vi "Terminate.vi"(8 "error in (no error)":errorcluster, 10 "Message in":refnum<class "TerminateMessage.lvclass">, 11 "Galvo in":refnum<class "ImagingModeSPIM.lvclass">) -> (0 "error out":errorcluster, 3 "Galvo out":refnum<class "ImagingModeSPIM.lvclass">)   [LabVIEW 2012, in "ImagingModeSPIM.lvclass"]
doc: "This member function is called when the statemachine in the run.vi receives an 'terminate' command. It closes the RabbitMQ connection. \n\nOverride this member function in your derived class to release all previously acquired resources (but don't forget to call the parent method). If your component has subcomponents, they count as resources, and you have to release them by calling their own terminate functions."
uses:
  ImagingModeSPIM.lvclass
  <vilib>/Distrio/Murmex/TerminateMessage/TerminateMessage.lvclass
  ImagingModeSPIM.lvclass/ImagingModeSPIM.ctl
  <vilib>/Distrio/Murmex/Murmex/Murmex.lvclass
panel:
  # "This method is called when the TERMINATE\ntrigger is sent. \n\nOverride this method when your component needs to\nrespond to this trigger. \n\nCall parent for proper implementation"
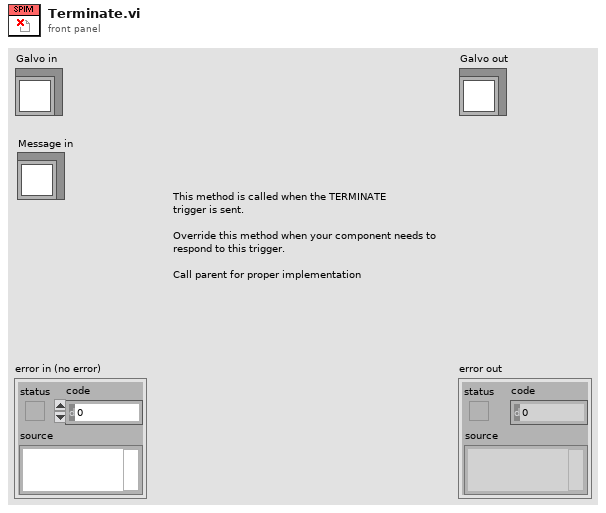
[diagram p1: front panel]
types:
  T1 = enum8{"Enabled", "Disabled", "Disabled and Grayed Out"}
  T2 = typedef "ImagingModeSPIM.lvclass/number of channels.ctl" = enum16{"empty", "double sided + PC", "double sided + WFS"}
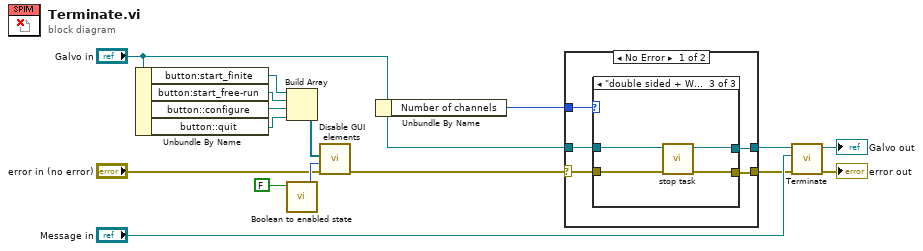
[diagram p0: block diagram]
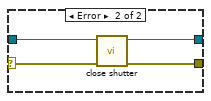
[diagram p4: hidden frame]
diagram:
  n1 = Unbundle By Name("Galvo in") -> ("button:start_finite"=w7:refnum<vi>, "button:start_free-run"=w8:refnum<vi>, "button::configure"=w9:refnum<vi>, "button::quit"=w10:refnum<vi>)
  n2 = Build Array(w7, w8, w9, w10) -> (w6:refnum<vi>[])
  n3 = call <vilib>:"Boolean to enabled state.vi"("boolean in"=FALSE) -> ("enabled status out"=w12:T1)  [unwired: 4 in]
  n4 = call <vilib>:"Disable GUI elements.vi"("error in (no error)"="error in (no error)", "enabled state"=w12, "control refs"=w6) -> ("error out"=w5:errorcluster)  [unwired: 8 in]
  n5 = Unbundle By Name("Galvo in") -> ("Number of channels"=w1:T2)
  n6 = case shown="No Error" w5 {
    selector: w5 -> [w21 w33]
    tunnel: [w20 w32] -> w4
    tunnel: "Galvo in" -> [w19 w31]
    tunnel: [w18 w30] -> w3
    tunnel: w1 -> [w17 _]
    frame No Error {
      n7 = case shown="\"double sided + WFS\"" w17 {
        tunnel: w21 -> [w22 w24 w28]
        tunnel: [w22 w24 w26] -> w20
        tunnel: w19 -> [w23 w25 w29]
        tunnel: [w23 w25 w27] -> w18
        frame "empty", Default {
        }
        frame "double sided + PC" {
        }
        frame "double sided + WFS" {
          n8 = call-dynamic "stop task.vi"("error in (no error)"=w28, "ImagingModeSPIM in"=w29) -> ("error out"=w26:errorcluster, "ImagingModeSPIM out"=w27:refnum<class "ImagingModeSPIM.lvclass">)  [unwired: 8 in]
        }
      }
    }
    frame Error {
      n9 = call "close shutter.vi"("error in (no error)"=w33, "Murmex in"=w31) -> ("error out"=w32:errorcluster, "Murmex out"=w30:refnum<class "ImagingModeSPIM.lvclass">)  [unwired: 8 in]
    }
  }
  n10 = call-parent "Terminate.vi"("error in (no error)"=w4, "Message in"="Message in", "Murmex in"=w3) -> ("error out"=→"error out":errorcluster, "Murmex out"=→"Galvo out":refnum<class "ImagingModeSPIM.lvclass">)  [unwired: 7 in]
